vi "Excit_Write_Wfm_Binary_Disk.vi"(7 "Excit Waveforms File Filter":string, 8 "error in (no error)":errorcluster, 9 "Waveform Name":string, 10 "Signal Excitation":dbl[](array[numeric]), 11 "Excit Waveforms Path":path) -> (0 "error out":errorcluster)   [LabVIEW 2017]
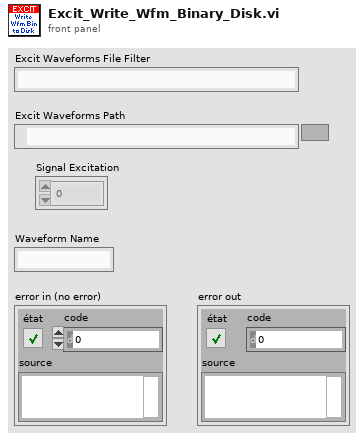
[diagram p1: front panel]
types:
  T1 = enum16{"open", "replace", "create", "open or create", "replace or create", "replace or create with confirmation"}
  T2 = enum16{"big-endian, network order", "native, host order", "little-endian"}
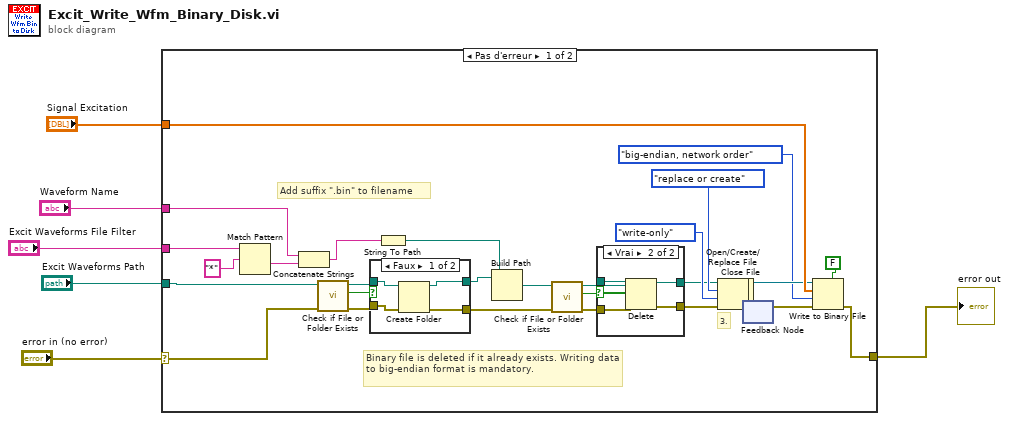
[diagram p0: block diagram]
diagram:
  n1 = case shown="Pas d'erreur" "error in (no error)" {
    selector: "error in (no error)" -> [w10 w48]
    tunnel: "Waveform Name" -> [w35 _]
    tunnel: "Excit Waveforms File Filter" -> [w31 _]
    tunnel: "Signal Excitation" -> [w30 _]
    tunnel: [w7 w48] -> w3
    tunnel: "Excit Waveforms Path" -> [w29 _]
    frame No Error {
      # "Binary file is deleted if it already exists. Writing data to big-endian format is mandatory."
      # "Add suffix \".bin\" to filename"
      # "3."
      n2 = Match Pattern(string=w31, regular expression="*" ("expression régulière")) -> (after substring=w33:string)  [unwired: 1 in, 3 out]
      n3 = Concatenate Strings(w35, w33) -> (w34:string)
      n4 = call <vilib>:"Check if File or Folder Exists.vi"("error in (no error)"=w10, "path"=w29) -> ("error out"=w13:errorcluster, "file or folder exists?"=w15:bool, "dup path"=w14:path)  [unwired: 7 in]
      n5 = case shown="Faux" w15 {
        tunnel: w14 -> [w39 w41]
        tunnel: [w38 w41] -> w12
        tunnel: w13 -> [w37 w40]
        tunnel: [w36 w40] -> w11
        frame False {
          n6 = Create Folder(path (use dialog)=w39, error in=w37) -> (created path=w38:path, error out=w36:errorcluster)  [unwired: 1 in, 1 out]
        }
        frame True {
        }
      }
      n7 = String To Path(string=w34) -> (path=w22:path)
      n8 = Build Path(base path=w12, name or relative path=w22) -> (appended path=w18:path)
      n9 = call <vilib>:"Check if File or Folder Exists.vi"("error in (no error)"=w11, "path"=w18) -> ("error out"=w19:errorcluster, "file or folder exists?"=w20:bool, "dup path"=w21:path)  [unwired: 7 in]
      n10 = case shown="Vrai" w20 {
        tunnel: w21 -> [w43 w47]
        tunnel: w19 -> [w42 w46]
        tunnel: [w43 w45] -> w17
        tunnel: [w42 w44] -> w16
        frame False {
        }
        frame True {
          n11 = Delete(path (use dialog)=w47, error in=w46) -> (deleted path=w45:path, error out=w44:errorcluster)  [unwired: 3 in, 1 out]
        }
      }
      n12 = Open/Create/Replace File(file path (use dialog)=w17, error in=w16, operation (0:open)=T1."replace or create", access (0:read/write)=enum16{"read/write", "read-only", "write-only"}."write-only") -> (refnum out=w27:refnum<file>)  [unwired: 2 in, 2 out]
      n13 = feedback #1() -> (w8:errorcluster)  [unwired: 1 in]
      n14 = Write to Binary File(file (use dialog)=w27, data=w30, error in=w8, 5:FALSE ("prepend array or string size? (T)"), 9:T2."big-endian, network order" ("byte order")) -> (refnum out=w28:refnum<file>, error out=w7:errorcluster)  [unwired: 1 in, 1 out]
      n15 = Close File(refnum=w28) -> (error out=w9:errorcluster)  [unwired: 1 in, 1 out]
      n16 = feedback-in #1(w9) -> ()
    }
    frame Error {
    }
  }
  "error out" <- w3
